vi "ModifyGraph grid.vi"(8 "error in (no error)":errorcluster, 11 "ITX Commands in":refnum<class "ITX Commands.lvclass">) -> (0 "error out":errorcluster, 3 "ITX Commands out":refnum<class "ITX Commands.lvclass">)   [LabVIEW 2019, in "ITX Commands.lvclass"]
uses:
  ITX Commands.lvclass
  ITX Commands.lvclass/ITX Commands.ctl
panel:
  out "resulting string":string
  in  "grid":string
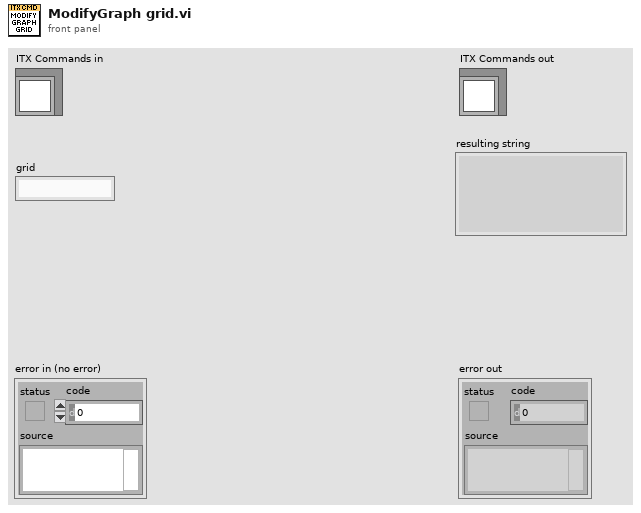
[diagram p1: front panel]
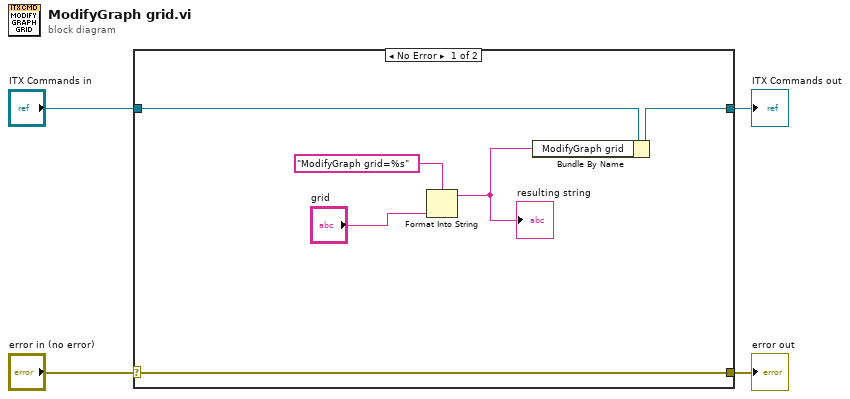
[diagram p0: block diagram]
diagram:
  n1 = case shown="No Error" "error in (no error)" {
    selector: "error in (no error)" -> [w10 w12]
    tunnel: [w10 w12] -> w3
    tunnel: [w8 w11] -> w1
    tunnel: "ITX Commands in" -> [w9 w11]
    frame No Error {
      n2 = Format Into String(format string="ModifyGraph grid=%s", "grid") -> (resulting string=w7:string)  [unwired: 2 in, 1 out]
      "resulting string" <- w7
      n3 = Bundle By Name(cluster=w9, "ModifyGraph grid"=w7) -> (w8:refnum<class "ITX Commands.lvclass">)
    }
    frame Error {
    }
  }
  "error out" <- w3
  "ITX Commands out" <- w1
